vi "SQLite Query - Select.vi"(6 "Column Value":string[](array[string])=["401", "q"], 7 "Columns Names":string[](array[string])=["Numeric Data", "String Data"], 8 "error in":errorcluster, 10 "Table Headers":string[](array[string]), 11 "Table Name":string) -> (0 "error out":errorcluster, 3 "SQLite Query":string)   [LabVIEW 2014, in "TableLogger_SQLite_Actor.lvlib" / "TableLogger_SQLite_Actor.lvclass"]
uses:
  TableLogger_SQLite_Actor.lvclass
  TableLogger_CSV_Actor/TableLogger_CSV_Actor/TableLogger_CSV_Actor.lvclass
panel:
  # "Numeric (Recnt)"
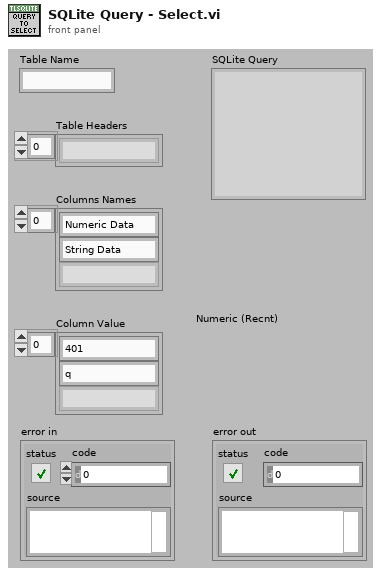
[diagram p1: front panel]
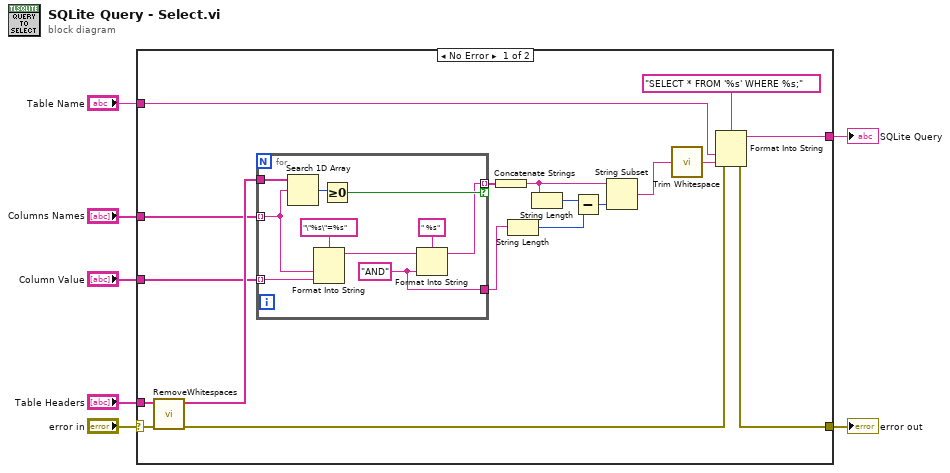
[diagram p0: block diagram]
diagram:
  n1 = case shown="No Error" "error in" {
    selector: "error in" -> [w24 w36]
    tunnel: "Table Name" -> [w22 _]
    tunnel: "Table Headers" -> [w25 _]
    tunnel: [w19 w36] -> w4
    tunnel: [w21 _] -> w3
    tunnel: "Columns Names" -> [w10 _]
    tunnel: "Column Value" -> [w9 _]
    frame No Error {
      n2 = call "RemoveWhitespaces.vi"("error in (no error)"=w24, "Array In"=w25) -> ("error out"=w20:errorcluster, "Array removing empty space"=w11:string[])  [unwired: 8 in]
      n3 = for {
        tunnel: w11 -> [w35]
        tunnel: w10 -> [w30] mode=indexing
        tunnel: w9 -> [w31] mode=indexing
        tunnel: [w28] -> w14 mode=indexing if=w33
        tunnel: [w26] -> w13
        w26 = "AND" ("input 1")
        n4 = Search 1D Array(1D array=w35, element=w30) -> (index of element=w34:i32)  [unwired: 1 in]
        n5 = Format Into String(format string="\"%s\"=%s", w30, w31) -> (resulting string=w29:string)  [unwired: 2 in, 1 out]
        n6 = Greater Or Equal To 0?(x=w34) -> (x >= 0?=w33:bool)
        n7 = Format Into String(format string=" %s", initial string=w29, w26) -> (resulting string=w28:string)  [unwired: 1 in, 1 out]
      }
      n8 = Concatenate Strings(w14) -> (w16:string)
      n9 = String Length(string=w13) -> (length=w12:i32)
      n10 = String Length(string=w16) -> (length=w17:i32)
      n11 = Subtract(x=w17, y=w12) -> (x-y=w18:i32)
      n12 = String Subset(string=w16, length (rest)=w18) -> (substring=w15:string)  [unwired: 1 in]
      n13 = call <vilib>:"Trim Whitespace.vi"("string"=w15) -> ("trimmed string"=w8:string)  [unwired: 1 in]
      n14 = Format Into String(format string="SELECT * FROM '%s' WHERE %s;" ("SQL"), error in=w20, w22, w8) -> (resulting string=w21:string, error out=w19:errorcluster)  [unwired: 1 in]
    }
    frame Error {
    }
  }
  "SQLite Query" <- w3
  "error out" <- w4
